vi "top.vi"() -> ()   [LabVIEW 2014]
panel:
  in  "?":cluster{bool, bool}
  # "SUDOKU"
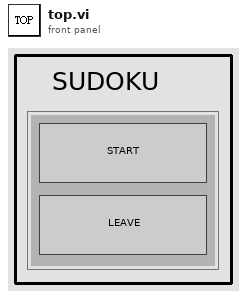
[diagram p1: front panel]
types:
  T1 = enum16{"wait bottum", "init", "start", "setting", "leave"}
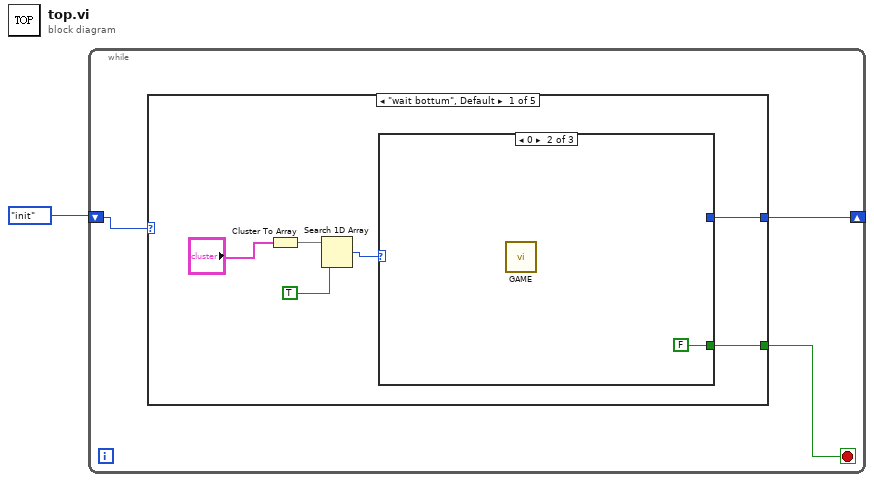
[diagram p0: block diagram]
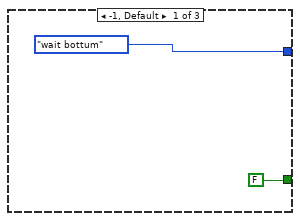
[diagram p2: hidden frame]
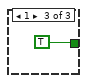
[diagram p3: hidden frame]
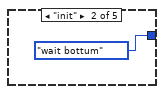
[diagram p4: hidden frame]
diagram:
  n1 = while {
    shift-right: [w3] -> _
    shift-left: T1."init" -> [w4]
    stop <- w2 stop-if-true
    n2 = case shown="\"wait bottum\", Default" w4 {
      tunnel: [w6 T1."wait bottum" _ _ _] -> w3
      tunnel: [w5 _ _ _ _] -> w2
      frame "wait bottum", Default {
        n3 = Cluster To Array(cluster="?") -> (array=w8:bool[])
        n4 = Search 1D Array(1D array=w8, element=TRUE) -> (index of element=w7:i32)  [unwired: 1 in]
        n5 = case shown="0" w7 {
          tunnel: [T1."wait bottum" _ _] -> w6
          tunnel: [FALSE FALSE TRUE] -> w5
          frame -1, Default {
          }
          frame 0 {
            n6 = call "GAME.vi"() -> ()  [unwired: 2 in]
          }
          frame 1 {
          }
        }
      }
      frame "init" {
      }
      frame "setting" {
      }
      frame "leave" {
      }
      frame "start" {
      }
    }
  }
